vi "Periodic Tasks.vi"(8 "error in":errorcluster) -> ()   [LabVIEW 2018]
doc: "This VI runs in parallel to other tasks. It can contain as many user-defined periodic loops as you need. These can carry out PID or other sorts of timed response."
uses:
  <vilib>/Rock Robotics/WPI/DriverStation/WPI_DriverStationRobotMode2.ctl
  <vilib>/Rock Robotics/WPI/Utilities/WPI_GetSetVariantRefNum.vi
  <vilib>/Rock Robotics/Network Tables/NT Read Number.vi
  Robot Global Data.vi
  <vilib>/Rock Robotics/Network Tables/NT Read Boolean.vi
  <vilib>/Rock Robotics/Network Tables/NT Write Numeric Array.vi
  <vilib>/Rock Robotics/Network Tables/NT Write Boolean Array.vi
  <vilib>/Rock Robotics/Network Tables/NT Write Number.vi
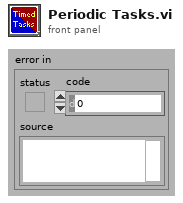
[diagram p1: front panel]
types:
  T1 = typedef "WPI_JoystickDevRef.ctl" = cluster{"Device":T2}
  T2 = typedef "WPI_JoystickDeviceEnum.ctl" = enum16{"USB 0", "USB 1", "USB 2", "USB 3", "USB 4", "USB 5"}
  T3 = typedef "WPI_RobotDriveDevRef.ctl" = cluster{"DevStatus":errorcluster, "Motors[]":T4[], "Square Inputs":bool, "Max Output":dbl}
  T4 = typedef "WPI_MotorControlDeviceRef.ctl" = cluster{"DeviceStatus":errorcluster, "Type":T5, "PWM":cluster{"PWM Channel":T6, "DeadBand":T7}, "CAN":cluster{"Device Number":u8, "SetOutput VI Ref":variant, "GetOutput VI Ref":variant, "Enable VI Ref":variant, "Disable VI Ref":variant, "Data":variant}, "Invert":bool, "DIO PWM":cluster{"PWM \"Enable\" Channel":T6, "DIOChannel":T8, "PWM Rate":dbl}}
  T5 = typedef "WPI_MotorControlType.ctl" = enum16{"PWM", "CAN", "DIO PWM"}
  T6 = typedef "FPGA_DIOPWMChannel.ctl" = enum8{"PWM 0", "PWM 1", "PWM 2", "PWM 3", "PWM 4", "PWM 5", "PWM 6", "PWM 7", "PWM 8", "PWM 9", "PWM MXP 0", "PWM MXP 1", "PWM MXP 2", "PWM MXP 3", "PWM MXP 4", "PWM MXP 5", "PWM MXP 6", "PWM MXP 7", "PWM MXP 8", "PWM MXP 9", "Invalid"}
  T7 = typedef "WPI_PWMDeadband.ctl" = cluster{"Name":string, "maxPositivePwm":i32, "minPositivePwm":i32, "centerPwm":i32, "maxNegativePwm":i32, "minNegativePwm":i32, "angularRange":u16}
  T8 = typedef "FPGA_DIOChannel.ctl" = enum8{"DIO 0", "DIO 1", "DIO 2", "DIO 3", "DIO 4", "DIO 5", "DIO 6", "DIO 7", "DIO 8", "DIO 9", "DIO MXP 0", "DIO MXP 1", "DIO MXP 2", "DIO MXP 3", "DIO MXP 4", "DIO MXP 5", "DIO MXP 6", "DIO MXP 7", "DIO MXP 8", "DIO MXP 9", "DIO MXP 10", "DIO MXP 11", "DIO MXP 12", "DIO MXP 13", "DIO MXP 14", "DIO MXP 15", "SPI Port CS1", "SPI Port CS2", "SPI Port CS3", "SPI Port MISO", "SPI Port MOSI", "Invalid"}
  T9 = typedef "WPI_GyroDevRef.ctl" = cluster{"DevStatus":errorcluster, "Analog Channel":T10, "Gain (VoltsPerDegree/Second)":dbl, "Gyro Type":enum16{"Analog", "XRS450"}, "Handle":i32, "SPI Bus":T11, "Device Found":bool, "Sample Rate":dbl, "Calibrate On Open":bool, "Offset":dbl}
  T10 = typedef "FPGA_AIChannel.ctl" = enum8{"AI 0", "AI 1", "AI 2", "AI 3", "AI MXP 0", "AI MXP 1", "AI MXP 2", "AI MXP 3", "Invalid"}
  T11 = typedef "spi_bus.ctl" = enum16{"SPI On-Board, CS0", "SPI On-Board, CS1", "SPI On-Board, CS2", "SPI On-Board, CS3", "SPI MXP", "Invalid"}
  T12 = cluster{"JoystickDevRef":T1, "JoystickDevRef":T1, "RobotDriveDevRef":T3, "GyroDevRef":T9}
  T13 = typedef "WPI_DriverStationRobotMode2.ctl" = enum16{"Autonomous Disabled", "Autonomous Enabled", "Teleop Disabled", "Teleop Enabled", "Disconnected", "Finish", "Test Disabled", "Test Enabled", "Emergency Stopped"}
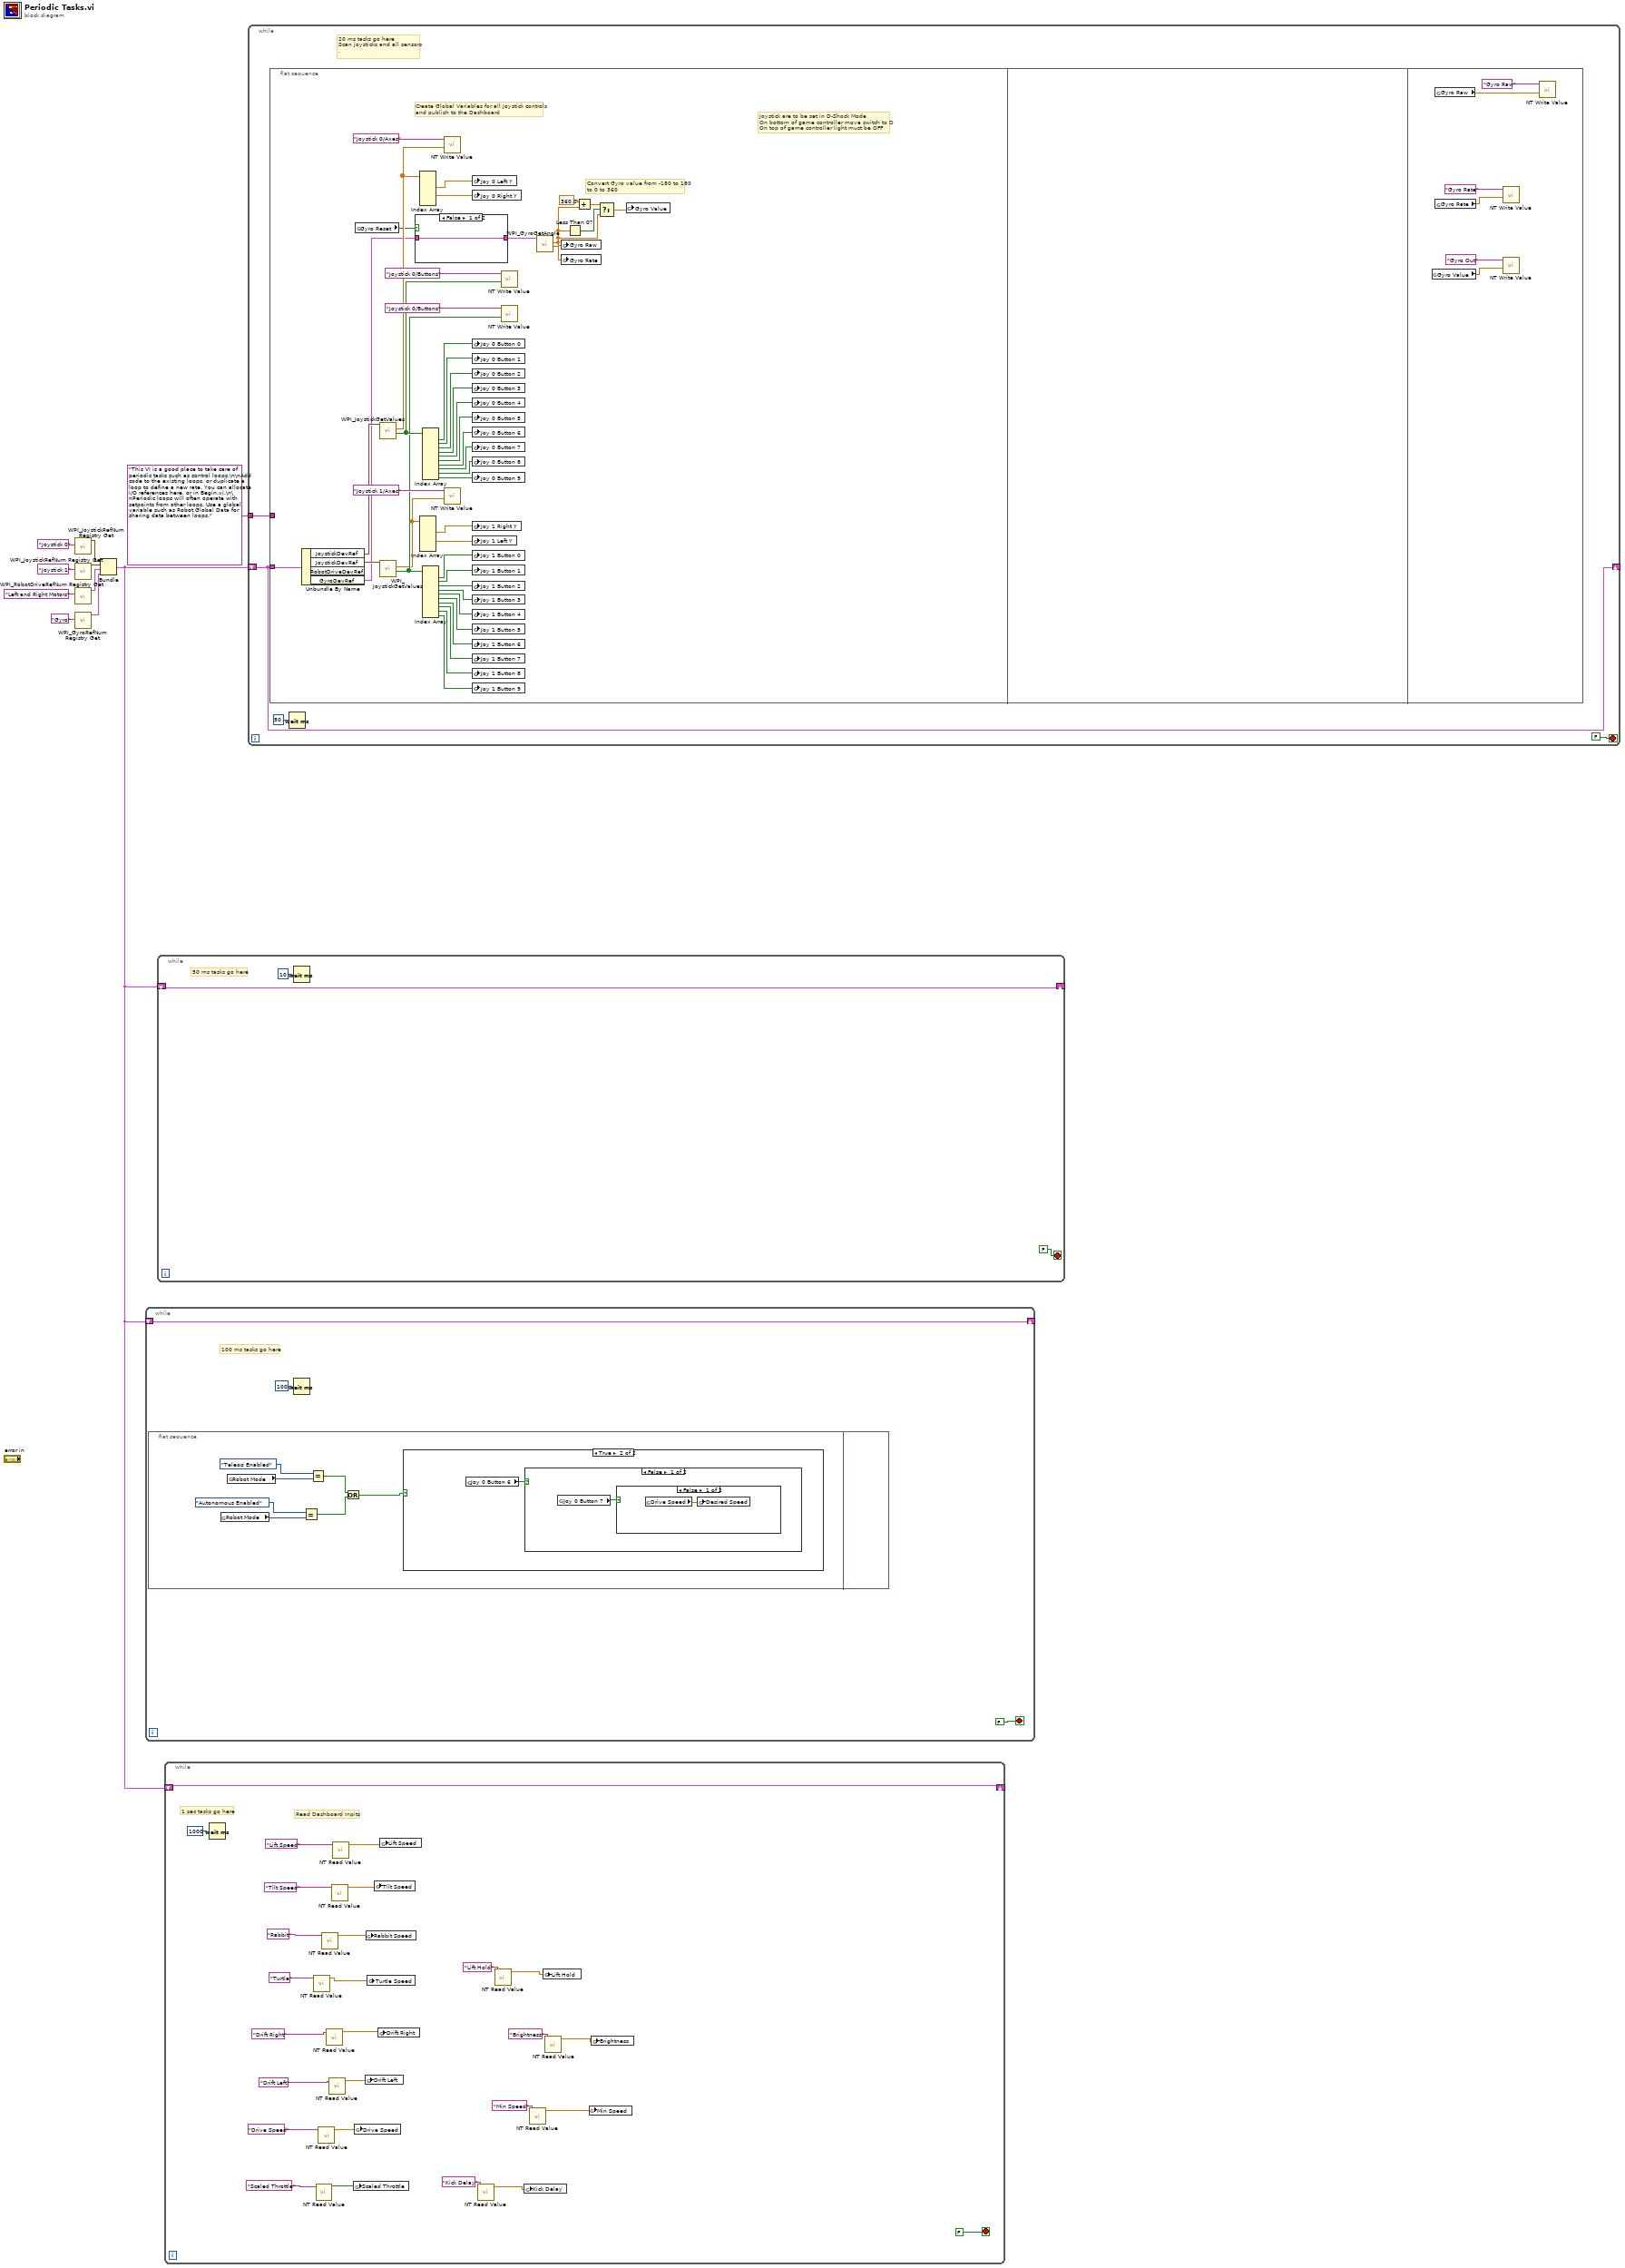
[diagram p0: block diagram]
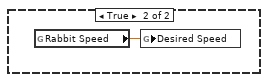
[diagram p3: hidden frame]
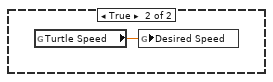
[diagram p4: hidden frame]
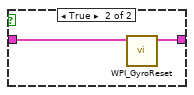
[diagram p5: hidden frame]
diagram:
  n1 = call <vilib>:"WPI_JoystickRefNum Registry Get.vi"("refnum name"="Joystick 0") -> ("JoystickDevRef"=w7:T1)  [unwired: 9 in, 1 out]
  n2 = call <vilib>:"WPI_JoystickRefNum Registry Get.vi"("refnum name"="Joystick 1") -> ("JoystickDevRef"=w4:T1)  [unwired: 9 in, 1 out]
  n3 = call <vilib>:"WPI_RobotDriveRefNum Registry Get.vi"("refnum name"="Left and Right Motors") -> ("RobotDriveDevRef"=w6:T3)  [unwired: 1 in, 9 out]
  n4 = call <vilib>:"WPI_GyroRefNum Registry Get.vi"("refnum name"="Gyro") -> ("GyroDevRef"=w3:T9)  [unwired: 9 in, 1 out]
  n5 = Bundle("JoystickDevRef"=w7, "JoystickDevRef"=w4, "RobotDriveDevRef"=w6, "GyroDevRef"=w3) -> (w2:T12)  [unwired: 1 out]
  n6 = while {
    shift-right: [w11] -> _
    shift-left: w2 -> [w11]
    stop <- FALSE stop-if-true
    # "100 ms tasks go here"
    n7 = flat-sequence {
      frame #0 {
        n8 = global read "Robot Global Data.vi" "Robot Mode"() -> (w18:T13)
        n9 = global read "Robot Global Data.vi" "Robot Mode"() -> (w20:T13)
        n10 = Equal?(x=WPI_DriverStationRobotMode2."Autonomous Enabled", y=w18) -> (x = y?=w14:bool)
        n11 = Equal?(x=WPI_DriverStationRobotMode2."Teleop Enabled", y=w20) -> (x = y?=w15:bool)
        n12 = Or(x=w15, y=w14) -> (x .or. y?=w16:bool)
        n13 = case shown="True" w16 {
          frame False {
          }
          frame True {
            n14 = global read "Robot Global Data.vi" "Joy 0 Button 6"() -> (w21:bool)
            n15 = case shown="False" w21 {
              frame False {
                n16 = global read "Robot Global Data.vi" "Joy 0 Button 7"() -> (w22:bool)
                n17 = case shown="False" w22 {
                  frame False {
                    n18 = global read "Robot Global Data.vi" "Drive Speed"() -> (w23:dbl)
                    n19 = global write "Robot Global Data.vi" "Desired Speed"(w23) -> ()
                  }
                  frame True {
                    n20 = global read "Robot Global Data.vi" "Rabbit Speed"() -> (w24:dbl)
                    n21 = global write "Robot Global Data.vi" "Desired Speed"(w24) -> ()
                  }
                }
              }
              frame True {
                n22 = global read "Robot Global Data.vi" "Turtle Speed"() -> (w25:dbl)
                n23 = global write "Robot Global Data.vi" "Desired Speed"(w25) -> ()
              }
            }
          }
        }
      }
      frame #1 {
      }
    }
    n24 = Wait (ms)(milliseconds to wait=u32 100) -> ()  [unwired: 1 out]
  }
  n25 = while {
    shift-right: [w26] -> _
    shift-left: w2 -> [w26]
    stop <- FALSE stop-if-true
    # "50 ms tasks go here"
    n26 = Wait (ms)(milliseconds to wait=u32 10) -> ()  [unwired: 1 out]
  }
  n27 = while {
    shift-right: [w53] -> _
    shift-left: w2 -> [w53]
    stop <- FALSE stop-if-true
    # "Read Dashboard Inpits"
    # "1 sec tasks go here"
    n28 = Wait (ms)(milliseconds to wait=u32 1000) -> ()  [unwired: 1 out]
    n29 = call-poly <vilib>:"NT Read Value.vi"("Name"="Turtle") -> ("Numeric"=w35:dbl)  [unwired: 9 in, 1 out]
    n30 = call-poly <vilib>:"NT Read Value.vi"("Name"="Scaled Throttle") -> ("Boolean"=w46:bool)  [unwired: 9 in, 1 out]
    n31 = call-poly <vilib>:"NT Read Value.vi"("Name"="Drive Speed") -> ("Numeric"=w33:dbl)  [unwired: 9 in, 1 out]
    n32 = call-poly <vilib>:"NT Read Value.vi"("Name"="Rabbit") -> ("Numeric"=w38:dbl)  [unwired: 9 in, 1 out]
    n33 = call-poly <vilib>:"NT Read Value.vi"("Name"="Drift Right") -> ("Numeric"=w34:dbl)  [unwired: 9 in, 1 out]
    n34 = call-poly <vilib>:"NT Read Value.vi"("Name"="Drift Left") -> ("Numeric"=w32:dbl)  [unwired: 9 in, 1 out]
    n35 = call-poly <vilib>:"NT Read Value.vi"("Name"="Tilt Speed") -> ("Numeric"=w36:dbl)  [unwired: 9 in, 1 out]
    n36 = call-poly <vilib>:"NT Read Value.vi"("Name"="Lift Speed") -> ("Numeric"=w37:dbl)  [unwired: 9 in, 1 out]
    n37 = global write "Robot Global Data.vi" "Scaled Throttle"(w46) -> ()
    n38 = global write "Robot Global Data.vi" "Drive Speed"(w33) -> ()
    n39 = global write "Robot Global Data.vi" "Drift Left"(w32) -> ()
    n40 = global write "Robot Global Data.vi" "Rabbit Speed"(w38) -> ()
    n41 = global write "Robot Global Data.vi" "Turtle Speed"(w35) -> ()
    n42 = global write "Robot Global Data.vi" "Tilt Speed"(w36) -> ()
    n43 = global write "Robot Global Data.vi" "Drift Right"(w34) -> ()
    n44 = global write "Robot Global Data.vi" "Lift Speed"(w37) -> ()
    n45 = call-poly <vilib>:"NT Read Value.vi"("Name"="Kick Delay") -> ("Numeric"=w42:dbl)  [unwired: 9 in, 1 out]
    n46 = call-poly <vilib>:"NT Read Value.vi"("Name"="Lift Hold") -> ("Numeric"=w29:dbl)  [unwired: 9 in, 1 out]
    n47 = global write "Robot Global Data.vi" "Kick Delay"(w42) -> ()
    n48 = call-poly <vilib>:"NT Read Value.vi"("Name"="Min Speed") -> ("Numeric"=w31:dbl)  [unwired: 9 in, 1 out]
    n49 = global write "Robot Global Data.vi" "Lift Hold"(w29) -> ()
    n50 = call-poly <vilib>:"NT Read Value.vi"("Name"="Brightness") -> ("Numeric"=w39:dbl)  [unwired: 9 in, 1 out]
    n51 = global write "Robot Global Data.vi" "Min Speed"(w31) -> ()
    n52 = global write "Robot Global Data.vi" "Brightness"(w39) -> ()
  }
  n53 = while {
    shift-right: [w57] -> _
    shift-left: w2 -> [w57]
    tunnel: "This VI is a good place to take care of periodic tasks such as control loops.\n\nAdd code to the existing loops, or duplicate a loop to define a new rate. You can allocate I/O references here, or in Begin.vi.\n\nPeriodic loops will often operate with setpoints from other loops. Use a global variable such as Robot Global Data for sharing data between loops." -> [w56]
    stop <- FALSE stop-if-true
    # "20 ms tasks go here\nScan joysticks and all sensors\n."
    n54 = flat-sequence {
      tunnel: w57 -> [w97]
      tunnel: w56 -> [_]
      frame #0 {
        # "Create Global Variables for all Joystick controls\nand publish to the Dashboard"
        # "Convert Gyro value from -180 to 180\nto 0 to 360"
        # "Joystick are to be set in D-Shock Mode\nOn bottom of game controller move switch to D\nOn top of game controller light must be OFF"
        n55 = Unbundle By Name(w97) -> ("JoystickDevRef"=w96:T1, "JoystickDevRef"=w81:T1, "GyroDevRef"=w66:T9)  [unwired: 1 out]
        n56 = global read "Robot Global Data.vi" "Gyro Reset"() -> (w65:bool)
        n57 = call <vilib>:"WPI_JoystickGetValues.vi"("JoystickDevRef"=w96) -> ("Buttons"=w90:bool[], "Axes"=w93:dbl[])  [unwired: 6 in, 3 out]
        n58 = call <vilib>:"WPI_JoystickGetValues.vi"("JoystickDevRef"=w81) -> ("Buttons"=w76:bool[], "Axes"=w60:dbl[])  [unwired: 6 in, 3 out]
        n59 = case shown="False" w65 {
          tunnel: [w104 w106] -> w67
          tunnel: w66 -> [w104 w105]
          frame False {
          }
          frame True {
            n60 = call <vilib>:"WPI_GyroReset.vi"("GyroDevRef"=w105) -> ("GyroDevRef"=w106:T9)  [unwired: 9 in, 1 out]
          }
        }
        n61 = Index Array(array=w93) -> (element #2=w92:dbl, element #4=w91:dbl)  [unwired: 6 in, 4 out]
        n62 = Index Array(array=w60) -> (element #2=w78:dbl, element #4=w79:dbl)  [unwired: 6 in, 4 out]
        n63 = Index Array(array=w90) -> (element #1=w89:bool, element #2=w88:bool, element #3=w87:bool, element #4=w86:bool, element #5=w85:bool, element #6=w84:bool, element #7=w83:bool, element #8=w82:bool, element #9=w62:bool, element #10=w61:bool)  [unwired: 10 in]
        n64 = Index Array(array=w76) -> (element #1=w75:bool, element #2=w74:bool, element #3=w73:bool, element #4=w72:bool, element #5=w71:bool, element #6=w70:bool, element #7=w69:bool, element #8=w68:bool, element #9=w64:bool, element #10=w63:bool)  [unwired: 10 in]
        n65 = call-poly <vilib>:"NT Write Value.vi"("Numeric Array"=w93, "Name"="Joystick 0/Axes") -> ()  [unwired: 9 in, 1 out]
        n66 = call-poly <vilib>:"NT Write Value.vi"("Numeric Array"=w60, "Name"="Joystick 1/Axes") -> ()  [unwired: 9 in, 1 out]
        n67 = global write "Robot Global Data.vi" "Joy 0 Left Y"(w92) -> ()
        n68 = global write "Robot Global Data.vi" "Joy 0 Right Y"(w91) -> ()
        n69 = global write "Robot Global Data.vi" "Joy 0 Button 0"(w89) -> ()
        n70 = global write "Robot Global Data.vi" "Joy 0 Button 1"(w88) -> ()
        n71 = global write "Robot Global Data.vi" "Joy 0 Button 2"(w87) -> ()
        n72 = global write "Robot Global Data.vi" "Joy 0 Button 3"(w86) -> ()
        n73 = global write "Robot Global Data.vi" "Joy 0 Button 4"(w85) -> ()
        n74 = global write "Robot Global Data.vi" "Joy 0 Button 5"(w84) -> ()
        n75 = global write "Robot Global Data.vi" "Joy 0 Button 6"(w83) -> ()
        n76 = global write "Robot Global Data.vi" "Joy 0 Button 7"(w82) -> ()
        n77 = global write "Robot Global Data.vi" "Joy 0 Button 8"(w62) -> ()
        n78 = global write "Robot Global Data.vi" "Joy 0 Button 9"(w61) -> ()
        n79 = global write "Robot Global Data.vi" "Joy 1 Right Y"(w78) -> ()
        n80 = global write "Robot Global Data.vi" "Joy 1 Left Y"(w79) -> ()
        n81 = global write "Robot Global Data.vi" "Joy 1 Button 0"(w75) -> ()
        n82 = global write "Robot Global Data.vi" "Joy 1 Button 1"(w74) -> ()
        n83 = global write "Robot Global Data.vi" "Joy 1 Button 2"(w73) -> ()
        n84 = global write "Robot Global Data.vi" "Joy 1 Button 3"(w72) -> ()
        n85 = global write "Robot Global Data.vi" "Joy 1 Button 4"(w71) -> ()
        n86 = global write "Robot Global Data.vi" "Joy 1 Button 5"(w70) -> ()
        n87 = global write "Robot Global Data.vi" "Joy 1 Button 6"(w69) -> ()
        n88 = global write "Robot Global Data.vi" "Joy 1 Button 7"(w68) -> ()
        n89 = global write "Robot Global Data.vi" "Joy 1 Button 8"(w64) -> ()
        n90 = global write "Robot Global Data.vi" "Joy 1 Button 9"(w63) -> ()
        n91 = call-poly <vilib>:"NT Write Value.vi"("Boolean Array"=w90, "Name"="Joystick 0/Buttons") -> ()  [unwired: 9 in, 1 out]
        n92 = call-poly <vilib>:"NT Write Value.vi"("Boolean Array"=w76, "Name"="Joystick 0/Buttons") -> ()  [unwired: 9 in, 1 out]
        n93 = call <vilib>:"WPI_GyroGetAngle.vi"("GyroDevRef"=w67) -> ("Angular Rate"=w99:dbl, "Angle"=w98:dbl)  [unwired: 6 in, 3 out]
        n94 = global write "Robot Global Data.vi" "Gyro Raw"(w98) -> ()
        n95 = global write "Robot Global Data.vi" "Gyro Rate"(w99) -> ()
        n96 = Less Than 0?(x=w98) -> (x < 0?=w102:bool)
        n97 = Add(x=360.0 ("y"), y=w98) -> (x+y=w101:dbl)
        n98 = Select(t=w101, s=w102, f=w98) -> (s? t:f=w103:dbl)
        n99 = global write "Robot Global Data.vi" "Gyro Value"(w103) -> ()
      }
      frame #1 {
      }
      frame #2 {
        n100 = global read "Robot Global Data.vi" "Gyro Value"() -> (w111:dbl)
        n101 = global read "Robot Global Data.vi" "Gyro Raw"() -> (w110:dbl)
        n102 = global read "Robot Global Data.vi" "Gyro Rate"() -> (w107:dbl)
        n103 = call-poly <vilib>:"NT Write Value.vi"("Numeric"=w107, "Name"="Gyro Rate") -> ()  [unwired: 9 in, 1 out]
        n104 = call-poly <vilib>:"NT Write Value.vi"("Numeric"=w111, "Name"="Gyro Out") -> ()  [unwired: 9 in, 1 out]
        n105 = call-poly <vilib>:"NT Write Value.vi"("Numeric"=w110, "Name"="Gyro Raw") -> ()  [unwired: 9 in, 1 out]
      }
    }
    n106 = Wait (ms)(milliseconds to wait=u32 50) -> ()  [unwired: 1 out]
  }
